vi "getLHeLevel.vi"(8 "error in (no error)":errorcluster, 11 "Instrument.Cryostat in":refnum<class "Instrument.Cryostat.lvclass">) -> (0 "error out":errorcluster, 2 "LHe Level (%)":dbl, 3 "Instrument.Cryostat out":refnum<class "Instrument.Cryostat.lvclass">)   [LabVIEW 2019, in "Instrument.Cryostat.lvclass"]
uses:
  Instrument.Cryostat.lvclass
  Typedefs/Cryostat.commands--enum.ctl
  d90b4709-2cc6-4655-808c-8eea05b18118.vi
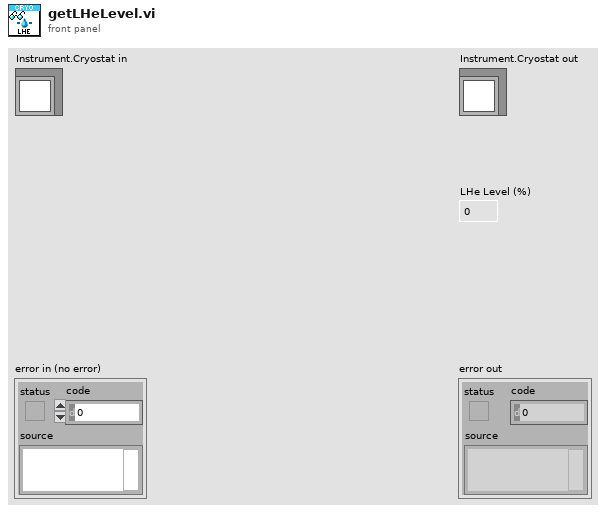
[diagram p1: front panel]
types:
  T1 = typedef "Instrument.Cryostat.lvclass/Cryostat.commands--enum.ctl" = enum16{"getLN2Level", "getLHeLevel", "getMagnet", "getMagnetVector", "setMagnet", "setMagnetVector", "getAngle", "setAngle", "getTemperature", "setTemperature", "getHeater", "setHeater", "getChamber", "setChamber", "getPressure"}
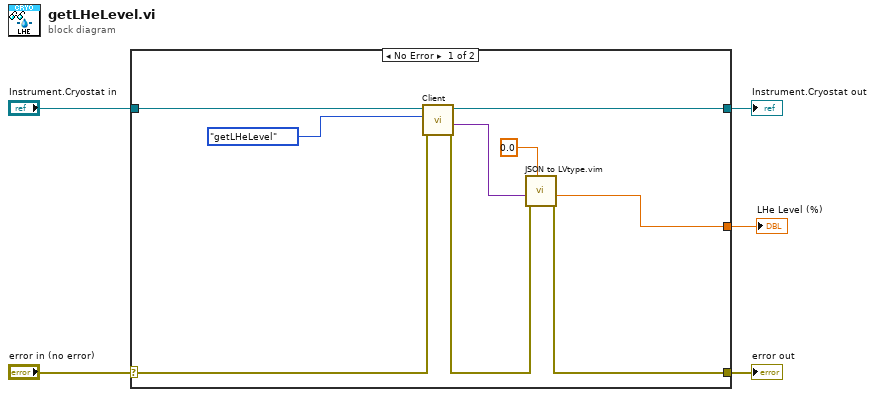
[diagram p0: block diagram]
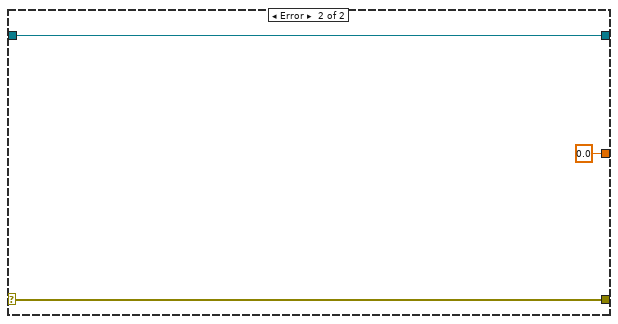
[diagram p2: hidden frame]
diagram:
  n1 = case shown="No Error" "error in (no error)" {
    selector: "error in (no error)" -> [w11 w17]
    tunnel: [w6 w17] -> w4
    tunnel: [w14 w16] -> w2
    tunnel: "Instrument.Cryostat in" -> [w13 w16]
    tunnel: [w7 0.0 ("Data out")] -> w1
    frame No Error {
      n2 = call-dynamic "Client.vi"("error in (no error)"=w11, "Command in"=Cryostat.commands--enum."getLHeLevel" ("commands"), "Instrument in"=w13) -> ("error out"=w8:errorcluster, "Data out"=w9:variant, "Instrument out"=w14:refnum<class "Instrument.Cryostat.lvclass">)  [unwired: 5 in, 1 out]
      n3 = call "JSON to LVtype.vim"("type"=0.0, "error in (no error)"=w8, "JSON Data in"=w9) -> ("error out"=w6:errorcluster, "Data out"=w7:dbl)  [unwired: 7 in]
    }
    frame Error {
    }
  }
  "error out" <- w4
  "Instrument.Cryostat out" <- w2
  "LHe Level (%)" <- w1
